vi "ActMakeTrajectory.vi"(8 "Max Speed":dbl, 9 "Initial Waypoint":T7={"X"=15.0, "Y"=105.0, "ANGLE"=-45.0, "WEIGHT"=2.0} {"WEIGHT" format="%13.3f"; "ANGLE" format="%13.3f"; "Y" format="%13.3f"; "X" format="%13.3f"}, 10 "Destination Waypoint":T7={"X"=210.0, "Y"=106.0, "ANGLE"=45.0, "WEIGHT"=2.0} {"WEIGHT" format="%13.3f"; "ANGLE" format="%13.3f"; "Y" format="%13.3f"; "X" format="%13.3f"}) -> (0 "Absolute Trajectory":T1 {"States"."POSE"."ROTATION"."SIN" format="%13.4f"; "States"."POSE"."ROTATION"."COS" format="%13.4f"; "States"."POSE"."ROTATION"."VALUE" format="%13.4f"; "States"."POSE"."TRANSLATION"."Y" format="%14.3f"; "States"."POSE"."TRANSLATION"."X" format="%14.3f"; "TotalTImeSecs" format="%20.3f"}, 1 "TotalTImeSecs":dbl, 2 "Trajectory Items":i32, 3 "Trajectory  creation error":errorcluster)   [LabVIEW 2023]
uses:
  <vilib>/Rock Robotics/WPI/ThirdParty/JAS_Junk/TrajLib/TypeDef/DISPLAY_WEIGHTED_WAYPOINT.ctl
  <vilib>/Rock Robotics/WPI/ThirdParty/JAS_Junk/TrajLib/Enum/TRAJECTORY_SPLINE_TYPE_ENUM.ctl
  <vilib>/Rock Robotics/WPI/ThirdParty/JAS_Junk/TrajLib/TypeDef/TRAJECTORY.ctl
  <vilib>/Rock Robotics/WPI/ThirdParty/JAS_Junk/TrajLib/TypeDef/TRAJ_STATE.ctl
  <vilib>/Rock Robotics/WPI/ThirdParty/JAS_Junk/TrajLib/TypeDef/POSE2D.ctl
  <vilib>/Rock Robotics/WPI/ThirdParty/JAS_Junk/TrajLib/TypeDef/TRANSLATION2D.ctl
  <vilib>/Rock Robotics/WPI/ThirdParty/JAS_Junk/TrajLib/TypeDef/ROTATION2D.ctl
  <vilib>/Rock Robotics/WPI/ThirdParty/JAS_Junk/TrajLib/Conv_Deg_Radians.vi
  <vilib>/Rock Robotics/WPI/ThirdParty/JAS_Junk/TrajLib/Util_DispWeightedWaypoint_To_WeightedWayPoint.vi
  <vilib>/Rock Robotics/WPI/ThirdParty/JAS_Junk/TrajLib/CentripetalAccelConstraint_New.vi
  <vilib>/Rock Robotics/WPI/ThirdParty/JAS_Junk/TrajLib/TrajectoryConfig_AddConstraint.vi
  <vilib>/Rock Robotics/WPI/ThirdParty/JAS_Junk/TrajLib/SwerveDriveKinematicsConstraint_New.vi
  <vilib>/Rock Robotics/WPI/ThirdParty/JAS_Junk/TrajLib/Translation2d_Create.vi
  <vilib>/Rock Robotics/WPI/ThirdParty/JAS_Junk/TrajLib/Rotation2d_CreateAngle.vi
  <vilib>/Rock Robotics/WPI/ThirdParty/JAS_Junk/TrajLib/Trajectory_Library.lvlib
panel:
  in  "Spline Type":T6
  out "MaxAcceleration  M/S^2":dbl=1.3 format="%17.4f"
  out "MaxVelocity M/S":dbl=2.0 format="%17.4f"
  out "Max Cent Accel":dbl=1.0 format="%20.4f"
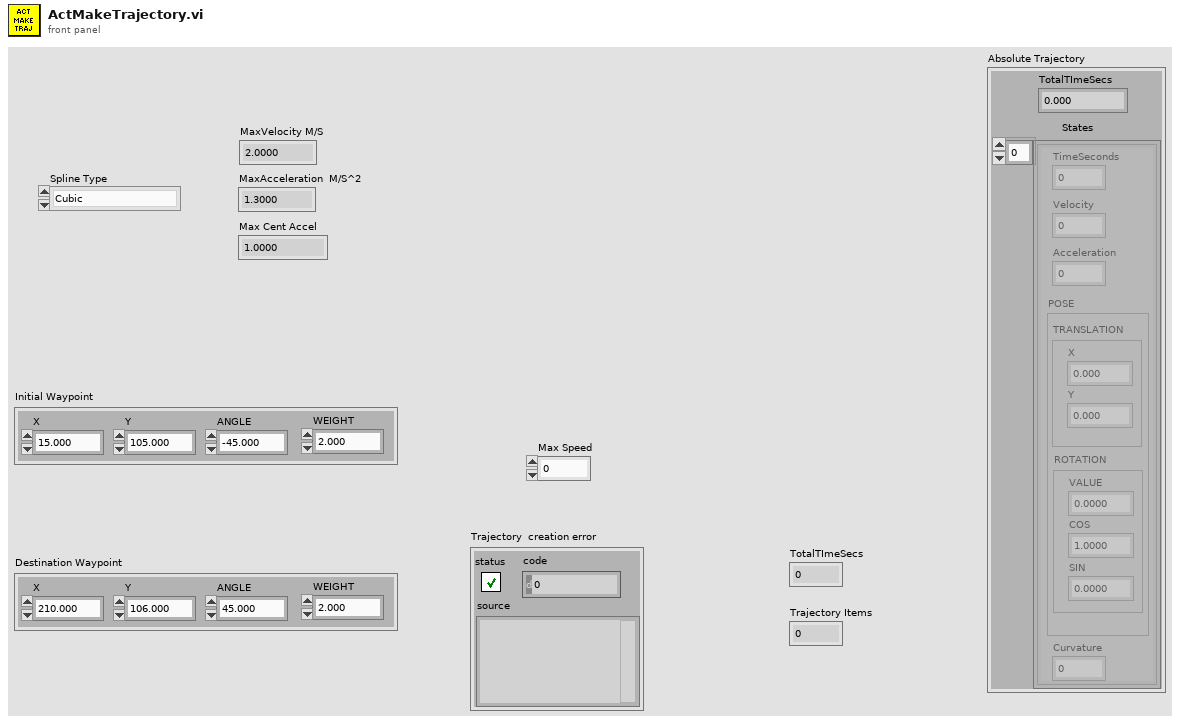
[diagram p1: front panel]
types:
  T1 = typedef "Trajectory_Library.lvlib/TRAJECTORY.ctl" = cluster{"TotalTImeSecs":dbl, "States":T2[]}
  T2 = typedef "Trajectory_Library.lvlib/TRAJ_STATE.ctl" = cluster{"TimeSeconds":dbl, "Velocity":dbl, "Acceleration":dbl, "POSE":T3, "Curvature":dbl}
  T3 = typedef "Trajectory_Library.lvlib/POSE2D.ctl" = cluster{"TRANSLATION":T4, "ROTATION":T5}
  T4 = typedef "Trajectory_Library.lvlib/TRANSLATION2D.ctl" = cluster{"X":dbl, "Y":dbl}
  T5 = typedef "Trajectory_Library.lvlib/ROTATION2D.ctl" = cluster{"VALUE":dbl, "COS":dbl, "SIN":dbl}
  T6 = typedef "Trajectory_Library.lvlib/TRAJECTORY_SPLINE_TYPE_ENUM.ctl" = enum16{"Cubic", "Cubic With Weights", "Quintic", "Quintic With Weights"}
  T7 = typedef "Trajectory_Library.lvlib/DISPLAY_WEIGHTED_WAYPOINT.ctl" = cluster{"X":dbl, "Y":dbl, "ANGLE":dbl, "WEIGHT":dbl}
  T8 = typedef "Trajectory_Library.lvlib/WEIGHTED_WAYPOINT.ctl" = cluster{"TRANSLATION":T4, "ROTATION":T5, "SCALAR":dbl}
  T9 = typedef "Trajectory_Library.lvlib/TRAJ_CONFIG.ctl" = cluster{"MaxVelocity":dbl, "Max Acceleration":dbl, "StartVelocity":dbl, "End Velocity":dbl, "Reversed":bool, "Constraints":variant[]}
  T10 = typedef "Trajectory_Library.lvlib/SWERVE_DRIVE_KINEMATICS.ctl" = cluster{"NumModules":i32, "InverseKinematics":T11, "ForwardKinematics":T11, "Modules":T4[], "PrevCoR":T4, "SavedModuleStates":T12[]}
  T11 = typedef "NI_Matrix.lvlib/RealMatrix.ctl" = dbl[][]
  T12 = typedef "Trajectory_Library.lvlib/SWERVE_DRIVE_MODULE_STATE.ctl" = cluster{"Speed":dbl, "Angle":T5}
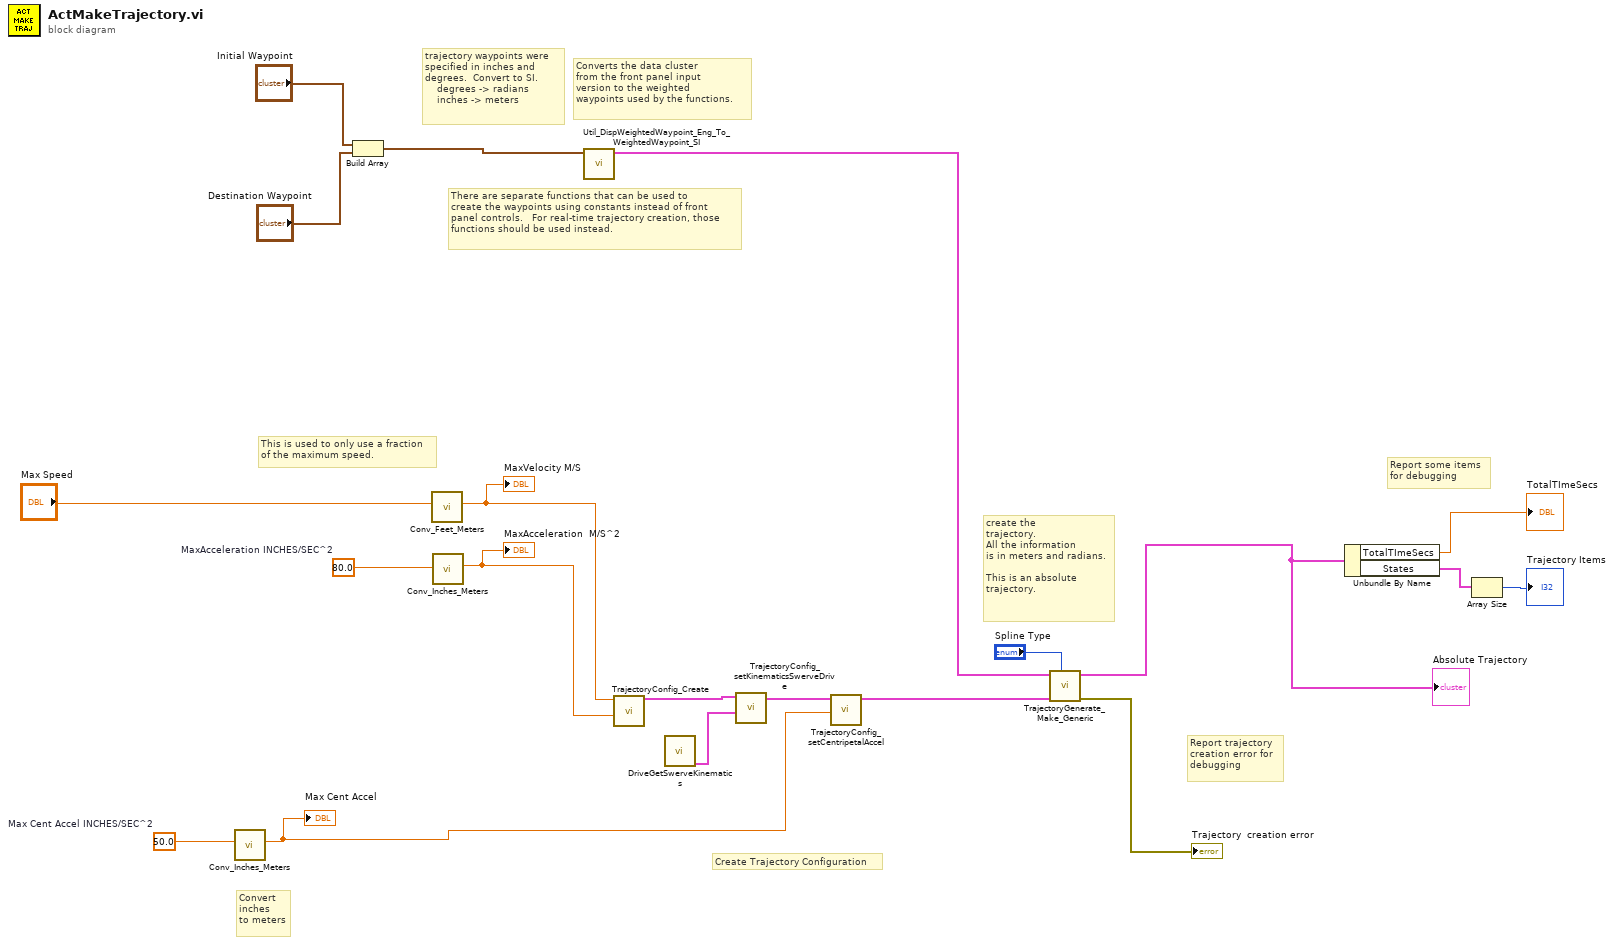
[diagram p0: block diagram]
diagram:
  w4 = 50.0  # Max Cent Accel INCHES/SEC^2
  w5 = 80.0  # MaxAcceleration INCHES/SEC^2
  # "There are separate functions that can be used to \ncreate the waypoints using constants instead of front\npanel controls.   For real-time trajectory creation, those\nfunctions should be used instead."
  # "This is used to only use a fraction\nof the maximum speed."
  # "Report trajectory\ncreation error for \ndebugging"
  # "Report some items\nfor debugging"
  # "Converts the data cluster\nfrom the front panel input\nversion to the weighted \nwaypoints used by the functions."
  # "Convert\ninches\nto meters"
  # "create the\ntrajectory.\nAll the information\nis in meters and radians.\n\nThis is an absolute \ntrajectory."
  # "trajectory waypoints were \nspecified in inches and\ndegrees.  Convert to SI.\n    degrees -> radians\n    inches -> meters"
  # "Create Trajectory Configuration"
  n1 = call <vilib>:"Conv_Inches_Meters.vi"("INCH"=w4) -> ("Meters"=w20:dbl)  [unwired: 10 in]
  "Max Cent Accel" <- w20
  n2 = Build Array("Initial Waypoint", "Destination Waypoint") -> (w10:T7[])
  n3 = call <vilib>:"Conv_Feet_Meters.vi"("Feet"="Max Speed") -> ("Meters"=w18:dbl)  [unwired: 10 in]
  "MaxVelocity M/S" <- w18
  n4 = call <vilib>:"Conv_Inches_Meters.vi"("INCH"=w5) -> ("Meters"=w19:dbl)  [unwired: 10 in]
  "MaxAcceleration  M/S^2" <- w19
  n5 = call <vilib>:"Util_DispWeightedWaypoint_Eng_To_WeightedWaypoint_SI.vi"("DisplayWeightedWayPoints_ENG"=w10) -> ("WeightedWayPoints_SI"=w9:T8[])  [unwired: 10 in]
  n6 = call <vilib>:"TrajectoryConfig_Create.vi"("MaxAcceleration"=w19, "MaxVelocity"=w18) -> ("TRAJECTORY_CONFIG"=w3:T9)  [unwired: 9 in]
  n7 = call "DriveGetSwerveKinematics.vi"() -> ("SWERVE_DRIVE_KINEMATICS"=w1:T10)  [unwired: 11 in]
  n8 = call <vilib>:"TrajectoryConfig_setKinematicsSwerveDrive.vi"("SWERVE_DRIVE_KINEMATICS"=w1, "inTRAJECTORY_CONFIG"=w3) -> ("outTRAJECTORY_CONFIG"=w2:T9)  [unwired: 9 in]
  n9 = call <vilib>:"TrajectoryConfig_setCentripetalAccel.vi"("Max Cent Accel"=w20, "inTRAJECTORY_CONFIG"=w2) -> ("outTRAJECTORY_CONFIG"=w16:T9)  [unwired: 9 in]
  n10 = call <vilib>:"TrajectoryGenerate_Make_Generic.vi"("Spline Type"="Spline Type", "traj_config"=w16, "WeightedWayPoints"=w9) -> ("error out"=→"Trajectory  creation error":errorcluster, "TRAJECTORY"=w8:T1)  [unwired: 7 in]
  "Absolute Trajectory" <- w8
  n11 = Unbundle By Name(w8) -> ("TotalTImeSecs"=→"TotalTImeSecs":dbl, "States"=w14:T2[])
  n12 = Array Size(array=w14) -> (size(s)=→"Trajectory Items":i32)
